vi "Create Column Definitions.vi"(8 "error in (no error)":errorcluster, 10 "Column":T1={"name"="", "caption"="", "datatype"=enum."string", "Params"="", "AutoSizeMode"=1, "FillWeight"=100.0, "MinWidth"=50, "tooltip"="", "ReadOnly?"=FALSE, "Visible?"=TRUE} {"MinWidth" min=2 step=1; "AutoSizeMode" items=["None"=1, "ColumnHeader"=2, "AllCellsExceptHeader"=4, "AllCells"=6, "DisplayedCellsExceptHeader"=8, "DisplayedCells"=10, "Fill"=16]; "FillWeight" min=1 max=100}) -> (0 "error out":errorcluster, 3 "GridColumn out":refnum<class "GridColumn.lvclass">)   [LabVIEW 2016, in "DataGrid.lvlib" / "GridColumn.lvclass"]
doc: "Based on the column inputs, the settings are applied to the .net TABLE column."
uses:
  <userlib>/LabVIEWdotNetDataGrid/source/GridColumn/GridColumn.lvclass
  <userlib>/LabVIEWdotNetDataGrid/source/GridColumn/ColumnDefinition.ctl
  <userlib>/LabVIEWdotNetDataGrid/source/GridColumn/ColumnType.ctl
  <userlib>/LabVIEWdotNetDataGrid/source/GridColumn/GridColumn.lvclass/GridColumn.ctl
  <userlib>/LabVIEWdotNetDataGrid/source/GridColumn/Write Name.vi
  <userlib>/LabVIEWdotNetDataGrid/source/GridColumn/Write datatype.vi
  <userlib>/LabVIEWdotNetDataGrid/source/GridColumn/Write Params.vi
  <userlib>/LabVIEWdotNetDataGrid/source/GridColumn/Write AutoSizeMode.vi
  <userlib>/LabVIEWdotNetDataGrid/source/GridColumn/Write Caption.vi
  <userlib>/LabVIEWdotNetDataGrid/source/GridColumn/Write Tooltip.vi
  <userlib>/LabVIEWdotNetDataGrid/source/GridColumn/Write ReadOnly.vi
  <userlib>/LabVIEWdotNetDataGrid/source/GridColumn/Write Visible.vi
  <userlib>/LabVIEWdotNetDataGrid/source/GridColumn/Write FillWeight.vi
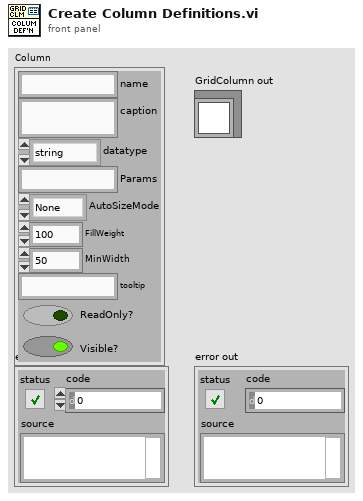
[diagram p1: front panel]
types:
  T1 = typedef "DataGrid.lvlib/GridColumn.lvclass/ColumnDefinition.ctl" = cluster{"name":string, "caption":string, "datatype":T2, "Params":string, "AutoSizeMode":i32, "FillWeight":sgl, "MinWidth":u32, "tooltip":string, "ReadOnly?":bool, "Visible?":bool}
  T2 = typedef "DataGrid.lvlib/GridColumn.lvclass/ColumnType.ctl" = enum16{"string", "image", "check", "numeric", "timestamp", "button", "combo", "link"}
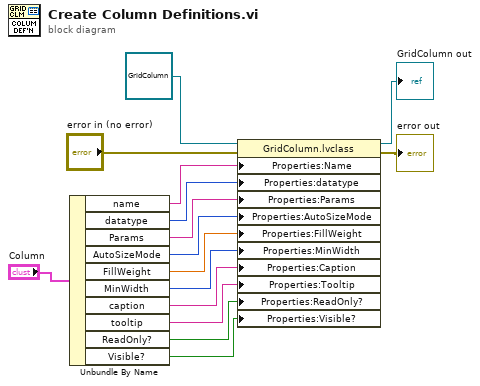
[diagram p0: block diagram]
diagram:
  n1 = Unbundle By Name("Column") -> ("name"=w12:string, "datatype"=w7:T2, "Params"=w13:string, "AutoSizeMode"=w14:i32, "FillWeight"=w15:sgl, "MinWidth"=w6:u32, "caption"=w4:string, "tooltip"=w3:string, "ReadOnly?"=w2:bool, "Visible?"=w1:bool)
  n2 = property class="GridColumn.lvclass"(reference=refnum<class "GridColumn.lvclass"> refnum ("GridColumn in"), error in="error in (no error)", "Properties:Name"=w12, "Properties:datatype"=w7, "Properties:Params"=w13, "Properties:AutoSizeMode"=w14, "Properties:FillWeight"=w15, "Properties:MinWidth"=w6, "Properties:Caption"=w4, "Properties:Tooltip"=w3, "Properties:ReadOnly?"=w2, "Properties:Visible?"=w1) -> (reference out=→"GridColumn out":refnum<class "GridColumn.lvclass">, error out=→"error out":errorcluster)
